vi "Read PZT File.vi"(11 "File Path Control":path) -> (3 "Layers":T1[](array[typedef]))   [LabVIEW 2022 SP3]
uses:
  Custom_Piezo.ctl
  PZT type.ctl
  <vilib>/Utility/file.llb/Read From Spreadsheet File (string).vi
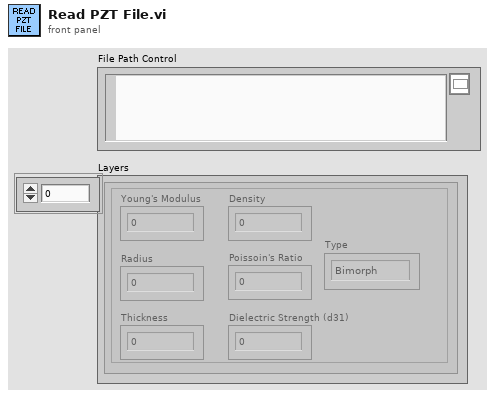
[diagram p1: front panel]
types:
  T1 = typedef "Custom_Piezo.ctl" = cluster{"Young's Modulus":dbl, "Radius":dbl, "Density":dbl, "Poissoin's Ratio":dbl, "Thickness":dbl, "Dielectric Strength (d31)":dbl, "Type":T2}
  T2 = typedef "PZT type.ctl" = enum16{"Bimorph", "Unimorph"}
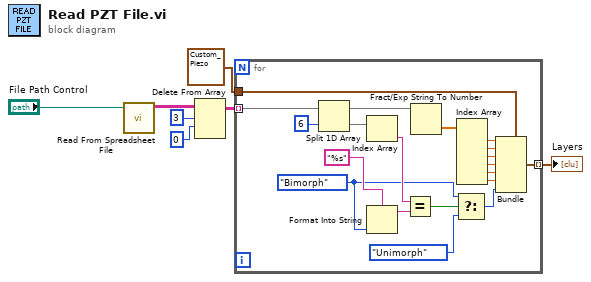
[diagram p0: block diagram]
diagram:
  n1 = call-poly <vilib>:"Read From Spreadsheet File.vi"("file path (dialog if empty)"="File Path Control") -> ("all rows"=w7:string[][])  [unwired: 6 in, 4 out]
  n2 = Delete From Array(array=w7, length=3, index (row)=0) -> (array with subset deleted=w4:string[][])  [unwired: 1 in, 1 out]
  n3 = for {
    tunnel: w4 -> [w27] mode=indexing
    tunnel: T1 {"Young's Modulus"=0.0, "Radius"=0.0, "Density"=0.0, "Poissoin's Ratio"=0.0, "Thickness"=0.0, "Dielectric Strength (d31)"=0.0, "Type"=enum."Unimorph"} ("Custom Piezo") -> [w18]
    tunnel: [w17] -> w2 mode=indexing
    w20 = PZT_type."Bimorph" ("Type")
    n4 = Split 1D Array(array=w27, index=6) -> (first subarray=w15:string[], second subarray=w25:string[])
    n5 = Index Array(array=w25) -> (element=w24:string)  [unwired: 1 in]
    n6 = Format Into String(format string="%s", w20) -> (resulting string=w22:string)  [unwired: 2 in, 1 out]
    n7 = Equal?(x=w24, y=w22) -> (x = y?=w21:bool)
    n8 = Fract/Exp String To Number(string=w15) -> (number=w14:dbl[])  [unwired: 3 in, 1 out]
    n9 = Select(t=w20, s=w21, f=PZT_type."Unimorph" ("Type")) -> (s? t:f=w16:T2)
    n10 = Index Array(array=w14) -> (element #1=w13:dbl, element #2=w12:dbl, element #3=w11:dbl, element #4=w10:dbl, element #5=w9:dbl, element #6=w8:dbl)  [unwired: 6 in]
    n11 = Bundle(cluster=w18, "Young's Modulus"=w13, "Radius"=w12, "Density"=w11, "Poissoin's Ratio"=w10, "Thickness"=w9, "Dielectric Strength (d31)"=w8, "Type"=w16) -> (w17:T1)
  }
  "Layers" <- w2
